vi "Extract Subclasses.vi"(10 "Base Class Name":string, 11 "Inheritance Map":T1) -> (2 "Subclass Names":string[](array[string]), 3 "Reduced Inheritance Map":T1)   [LabVIEW 2013]
uses:
  <userlib>/ICON Technologies/ICON Maps/lvlib/Map.ctl
  <userlib>/ICON Technologies/ICON Maps/lvlib/_Polymorphic Instances/Map_Value_Variant.vi
  <userlib>/ICON Technologies/ICON Maps/ICON Maps.lvlib
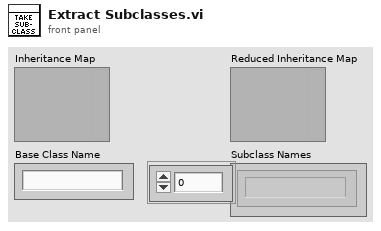
[diagram p1: front panel]
types:
  T1 = typedef "ICON Maps.lvlib/Map.ctl" = variant
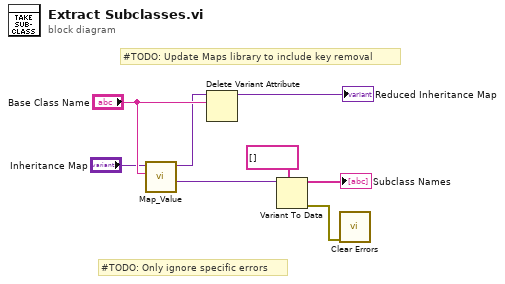
[diagram p0: block diagram]
diagram:
  # "#TODO: Only ignore specific errors"
  # "#TODO: Update Maps library to include key removal"
  n1 = call-poly <userlib>:"Map_Value.vi"("Key"="Base Class Name", "Map In"="Inheritance Map") -> ("Value"=w6:variant, "Map Out"=w2:T1)  [unwired: 8 in]
  n2 = Delete Variant Attribute(6:"Base Class Name", 7:w2) -> (3:→"Reduced Inheritance Map":variant)  [unwired: 1 in, 2 out]
  n3 = Variant To Data(type=string[] [] ("value 2"), Variant=w6) -> (data=→"Subclass Names":string[], error out=w4:errorcluster)  [unwired: 1 in]
  n4 = call <vilib>:"Clear Errors.vi"("error in (no error)"=w4) -> ()  [unwired: 6 in, 1 out]
